vi "Convert Output from Raw to FXP.vi"(7 "Relative Position":T1, 8 "error in (no error)":errorcluster, 9 "Term Refnum":refnum<vi>, 10 "Diagram":refnum<vi>, 11 "Signal in":refnum<class "Signal.lvclass">) -> (0 "error out":errorcluster, 1 "Term Refnum out":refnum<vi>, 3 "Signal out":refnum<class "Signal.lvclass">)   [LabVIEW 2025, in "Signal.lvclass"]
uses:
  Signal.lvclass
  <vilib>/_script/New VI Object TypeDefs/NewVIObject_LVRelativePositionTypeDef.ctl
  <vilib>/_script/New VI Object TypeDefs/NewVIObject_LVRelativeDirectionTypeDef.ctl
  <vilib>/Utility/miscctls.llb/LVPoint32TypeDef.ctl
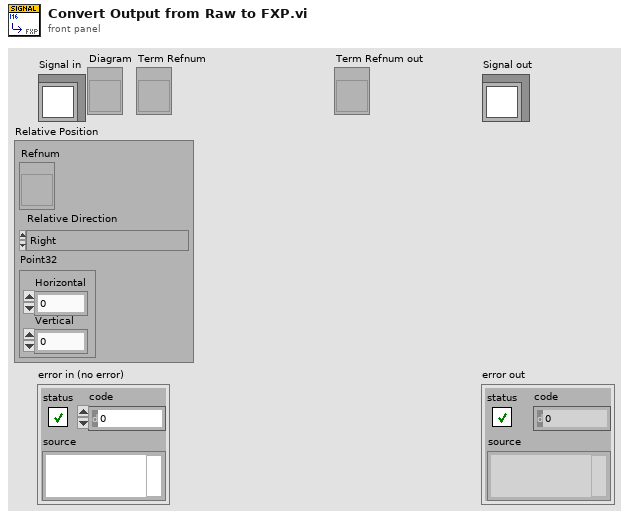
[diagram p1: front panel]
types:
  T1 = typedef "NewVIObject_LVRelativePositionTypeDef.ctl" = cluster{"Refnum":refnum<vi>, "Relative Direction":T2, "Point32":T3}
  T2 = typedef "NewVIObject_LVRelativeDirectionTypeDef.ctl" = enum32{"Right", "Left", "Top", "Bottom", "Top Right", "Top Left", "Bottom Right", "Bottom Left"}
  T3 = typedef "LVPoint32TypeDef.ctl" = cluster{"Horizontal":i32, "Vertical":i32}
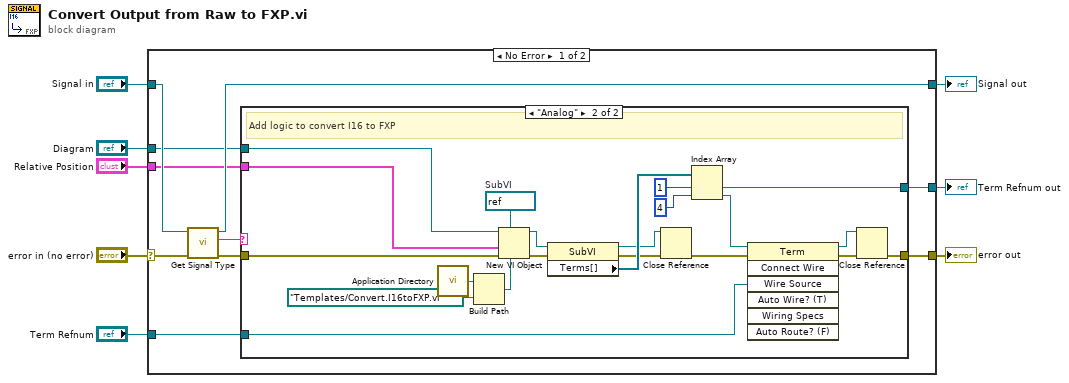
[diagram p0: block diagram]
diagram:
  n1 = case shown="No Error" "error in (no error)" {
    selector: "error in (no error)" -> [w16 w44]
    tunnel: [w15 w44] -> w7
    tunnel: [w13 w43] -> w5
    tunnel: "Signal in" -> [w14 w43]
    tunnel: "Diagram" -> [w12 _]
    tunnel: "Relative Position" -> [w11 _]
    tunnel: "Term Refnum" -> [w10 w42]
    tunnel: [w9 w42] -> w1
    frame No Error {
      n2 = call "Get Signal Type.vi"("error in (no error)"=w16, "IO Class in"=w14) -> ("error out"=w18:errorcluster, "Type"=w17:string, "IO Class out"=w13:refnum<class "Signal.lvclass">)  [unwired: 7 in]
      n3 = case shown="\"Analog\"" w17 {
        tunnel: w18 -> [w19 w40]
        tunnel: [w20 w29] -> w9
        tunnel: w10 -> [w20 w27]
        tunnel: w12 -> [_ w36]
        tunnel: w11 -> [_ w35]
        tunnel: [w19 w21] -> w15
        frame Default {
        }
        frame "Analog" {
          w41 = refnum<vi> refnum  # SubVI
          # "Add logic to convert I16 to FXP"
          n4 = call <vilib>:"Application Directory.vi"() -> ("Application Directory"=w39:path)
          n5 = Build Path(base path=w39, name or relative path=path "Templates/Convert.I16toFXP.vi" ("Application Directory")) -> (appended path=w37:path)
          n6 = New VI Object(vi object class=w41, owner refnum=w36, position/next to=w35, 6:w37, 8:w40) -> (object refnum=w33:refnum<vi>, 0:w34:errorcluster)  [unwired: 3 in]
          n7 = property class="SubVI"(reference=w33, error in=w34) -> (reference out=w22:refnum<vi>, error out=w24:errorcluster, "Terms[]"=w32:refnum<vi>[])
          n8 = Close Reference(reference=w22, error in (no error)=w24) -> (error out=w23:errorcluster)
          n9 = Index Array(array=w32, index #1=1 ("index"), index #2=4 ("index")) -> (element #1=w29:refnum<vi>, element #2=w28:refnum<vi>)
          n10 = invoke class="Term" method="Connect Wire"(reference=w28, error in=w23, "Wire Source"=w27) -> (reference out=w25:refnum<vi>, error out=w26:errorcluster)  [unwired: 4 in, 5 out]
          n11 = Close Reference(reference=w25, error in (no error)=w26) -> (error out=w21:errorcluster)
        }
      }
    }
    frame Error {
    }
  }
  "error out" <- w7
  "Signal out" <- w5
  "Term Refnum out" <- w1
